vi "callVNA.vi"   [LabVIEW 2019]
uses:
  <userlib>/LevyLab/Transport/Control Experiment/Control Experiment.lvclass/Control Experiment.ctl
  <userlib>/LevyLab/Transport/Transport/Transport.lvclass/Transport.ctl
  <userlib>/LevyLab/Transport/Transport/Transport.lvclass
  <userlib>/LevyLab/Transport/Control Experiment/Control Experiment.lvclass
  <vilib>/Wiresmith Technology/G CLI/CLI Class/CLI.lvclass
panel:
  # "[FLEX <-> VNA] \nThis VI calls VNA.vi upon a terminal command\ncommand: g-cli --lv-ver 2019 <path of the vi>"
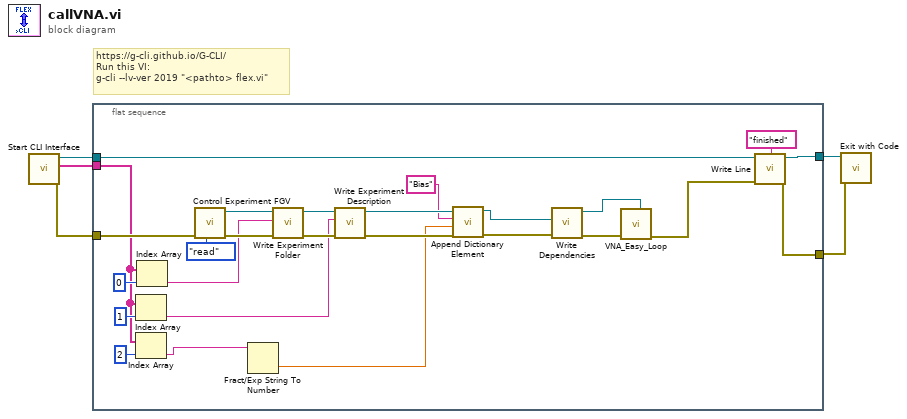
[diagram p0: block diagram]
diagram:
  # "https://g-cli.github.io/G-CLI/\nRun this VI:\ng-cli --lv-ver 2019 \"<pathto> flex.vi\""
  n1 = call <vilib>:"Start CLI Interface.vi"() -> ("error out"=w5:errorcluster, "Custom Parameters"=w1:string[], "CLI out"=w4:refnum<class "CLI.lvclass">)  [unwired: 8 in, 1 out]
  n2 = flat-sequence {
    tunnel: w5 -> [w30]
    tunnel: w4 -> [w28]
    tunnel: [w27] -> w3
    tunnel: [w26] -> w2
    tunnel: w1 -> [w8]
    frame #0 {
      n3 = Index Array(array=w8, index=1) -> (element=w15:string)
      n4 = Index Array(array=w8, index=2) -> (element=w7:string)
      n5 = Index Array(array=w8, index=0) -> (element=w18:string)
      n6 = call <userlib>:"Control Experiment FGV.vi"("Function"=enum16{"read", "write"}."read", "error in (no error)"=w30) -> ("error out"=w23:errorcluster, "Control Experiment.lvclass out"=w25:refnum<class "Control Experiment.lvclass">)  [unwired: 8 in]
      n7 = Fract/Exp String To Number(string=w7) -> (number=w6:dbl)  [unwired: 3 in, 1 out]
      n8 = call <userlib>:"Write Experiment Folder.vi"("error in (no error)"=w23, "Experiment Folder"=w18, "Control Experiment in"=w25) -> ("error out"=w22:errorcluster, "Control Experiment out"=w24:refnum<class "Control Experiment.lvclass">)  [unwired: 7 in]
      n9 = call <userlib>:"Write Experiment Description.vi"("error in (no error)"=w22, "Experiment Description"=w15, "Control Experiment in"=w24) -> ("error out"=w10:errorcluster, "Control Experiment out"=w12:refnum<class "Control Experiment.lvclass">)  [unwired: 7 in]
      n10 = call <userlib>:"Append Dictionary Element.vi"("error in (no error)"=w10, "value"=w6, "key"="Bias", "Control Experiment in"=w12) -> ("error out"=w13:errorcluster, "Control Experiment out"=w14:refnum<class "Control Experiment.lvclass">)  [unwired: 6 in]
      n11 = call <userlib>:"Write Dependencies.vi"("error in (no error)"=w13, "Control Experiment"=w14) -> ("error out"=w20:errorcluster, "Transport out"=w21:refnum<class "Transport.lvclass">)  [unwired: 8 in]
      n12 = call "VNA_Easy_Loop.vi"("Transport"=w21, "error in (no error)"=w20) -> ("error out"=w19:errorcluster)  [unwired: 8 in, 1 out]
      n13 = call <vilib>:"Write Line.vi"("error in (no error)"=w19, "Text to Write"="finished", "CLI in"=w28) -> ("error out"=w26:errorcluster, "CLI out"=w27:refnum<class "CLI.lvclass">)  [unwired: 7 in]
    }
  }
  n14 = call <vilib>:"Exit with Code.vi"("error in (no error)"=w2, "CLI in"=w3) -> ()  [unwired: 9 in, 1 out]
